vi "GEA2 Serial Get Bytes Data.vi"(6 "Bytes Data":u8[](array[numeric]), 7 "Current Read Index":i32, 8 "Error In":errorcluster, 9 "Bytes Remaining":u8, 10 "CRCArray":u8[](array[numeric]), 11 "ReadArray":u8[](array[numeric])) -> (0 "Error Out":errorcluster, 1 "Bytes Remaining":u8, 2 "CRC Array":u8[](array[numeric]), 3 "Current Read Index":i32, 4 "Bytes Data Out":u8[](array[numeric]), 5 "Parse Bytes":bool)   [LabVIEW 2014]
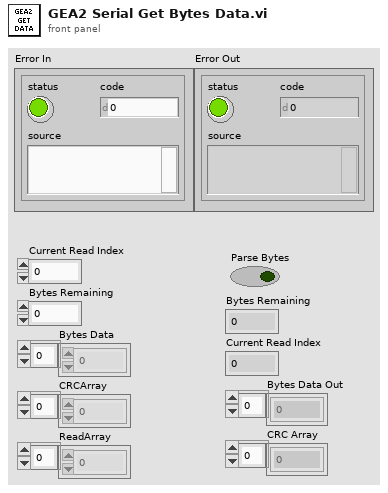
[diagram p1: front panel]
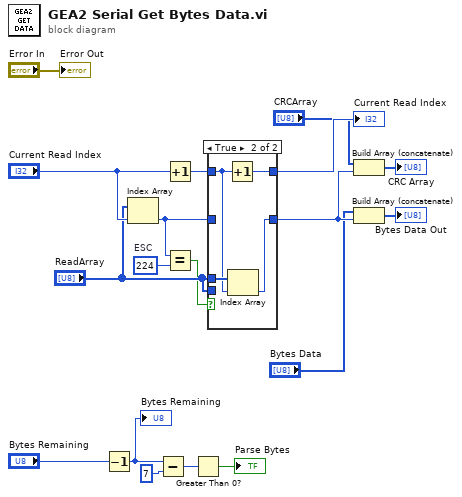
[diagram p0: block diagram]
diagram:
  w2 = u8 224  # ESC
  n1 = Decrement(x="Bytes Remaining") -> (x-1=w12:u8)
  "Bytes Remaining" <- w12
  n2 = Index Array(array="ReadArray", index="Current Read Index") -> (element=w18:u8)
  n3 = Subtract(x=w12, y=u8 7) -> (x-y=w14:u8)
  n4 = Increment(x="Current Read Index") -> (x+1=w17:i32)
  n5 = Equal?(x=w18, y=w2) -> (x = y?=w3:bool)
  n6 = Greater Than 0?(x=w14) -> (x > 0?=→"Parse Bytes":bool)
  n7 = case shown="True" w3 {
    tunnel: [w19 w21] -> w10
    tunnel: [w20 w24] -> w7
    tunnel: "ReadArray" -> [_ w23]
    tunnel: "ReadArray" -> [_ _]
    tunnel: w17 -> [w20 w22]
    tunnel: w18 -> [w19 _]
    frame False {
    }
    frame True {
      n8 = Increment(x=w22) -> (x+1=w24:i32)
      n9 = Index Array(array=w23, index=w22) -> (element=w21:u8)
    }
  }
  "Current Read Index" <- w7
  n10 = Build Array (concatenate)("CRCArray", w10) -> (→"CRC Array":u8[])
  n11 = Build Array (concatenate)("Bytes Data", w10) -> (→"Bytes Data Out":u8[])
  "Error Out" <- "Error In"
